vi "Detect and Decode Multiple (Greyscale).vi"(8 "error in (no error)":errorcluster, 10 "Greyscale Image in":T4, 11 "QR Code Detector in":refnum<class "QR Code Detector.lvclass">) -> (0 "error out":errorcluster, 2 "Detections":T1[](array[typedef]), 3 "QR Code Detector":refnum<class "QR Code Detector.lvclass">)   [LabVIEW 2020, in "feature_detection.lvlib" / "QR Code Detector.lvclass"]
doc: "Perform the Detection and Decoding steps on an Image which can contain multiple QR Codes."
uses:
  QR Code Detector.lvclass
  image/Greyscale Image.ctl
  Detection.ctl
  common/Image Points Quad (Float).ctl
  common/Image Point (Float).ctl
  QR Code Detector.lvclass/QR Code Detector.ctl
  97a01b78-84de-4c9d-a407-2dc45d320d5a.vi
  <vilib>/Utility/error.llb/Error Cluster From Error Code.vi
  image/image.lvlib
  common/common.lvlib
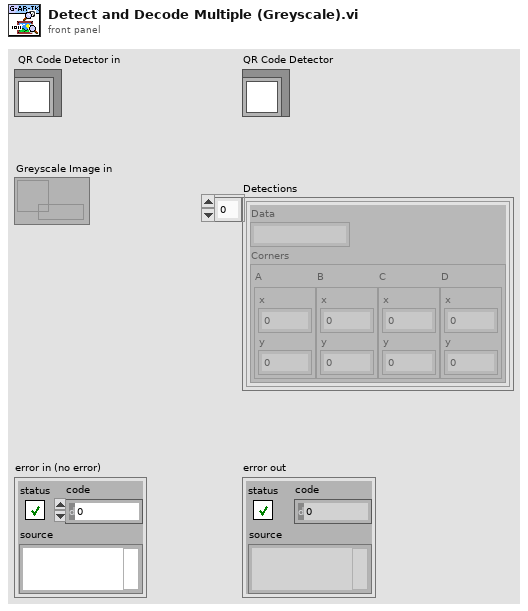
[diagram p1: front panel]
types:
  T1 = typedef "feature_detection.lvlib/QR Code Detector.lvclass/Detection.ctl" = cluster{"Data":string, "Corners":T2}
  T2 = typedef "common.lvlib/Image Points Quad (Float).ctl" = cluster{"A":T3, "B":T3, "C":T3, "D":T3}
  T3 = typedef "common.lvlib/Image Point (Float).ctl" = cluster{"x":dbl, "y":dbl}
  T4 = typedef "image.lvlib/Greyscale Image.ctl" = refnum<data-value>
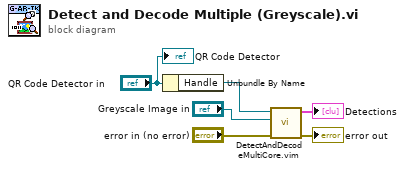
[diagram p0: block diagram]
diagram:
  n1 = Unbundle By Name("QR Code Detector in") -> ("Handle"=w1:refnum<data-value>)
  n2 = call "DetectAndDecodeMultiCore.vim"("error in (no error)"="error in (no error)", "Image"="Greyscale Image in", "Handle"=w1) -> ("error out"=→"error out":errorcluster, "Detections"=→"Detections":T1[])  [unwired: 7 in]
  "QR Code Detector" <- "QR Code Detector in"
